vi "stop.vi"(8 "error in (no error)":errorcluster, 11 "TaskController in":refnum<class "TaskController.lvclass">) -> (0 "error out":errorcluster, 3 "TaskController out":refnum<class "TaskController.lvclass">)   [LabVIEW 2023, in "TLC_Daemon.lvlib" / "TaskController.lvclass"]
doc: "Stops the task (waits the task to finish executing).\n_____________________________________\nTLC Daemon 1.0.0.2\nCopyright (c) 2026 Andrea Cadei"
uses:
  TaskController.lvclass
  TaskController.lvclass/TaskController.ctl
  ITaskStopMechanism/ITaskStopMechanism.lvclass
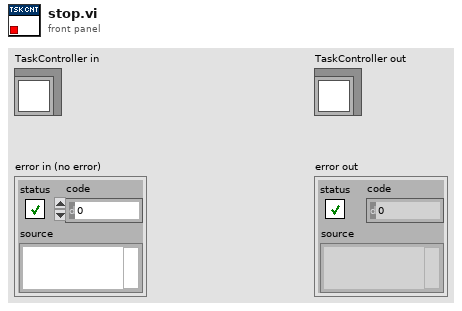
[diagram p1: front panel]
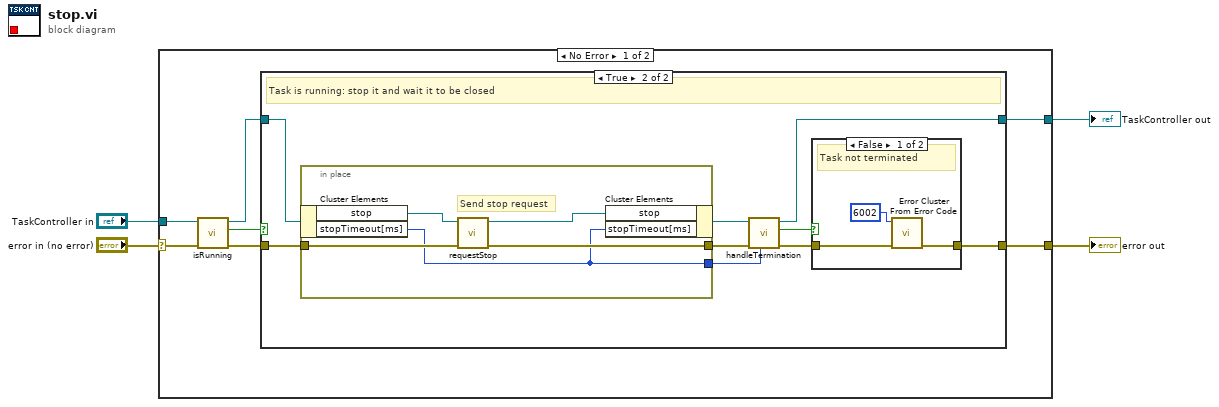
[diagram p0: block diagram]
diagram:
  n1 = case shown="No Error" "error in (no error)" {
    selector: "error in (no error)" -> [w7 w33]
    tunnel: [w10 w33] -> w3
    tunnel: [w11 w32] -> w1
    tunnel: "TaskController in" -> [w8 w32]
    frame No Error {
      n2 = call "isRunning.vi"("error in (no error)"=w7, "TaskController in"=w8) -> ("error out"=w6:errorcluster, "isRunning"=w5:bool, "TaskController out"=w9:refnum<class "TaskController.lvclass">)  [unwired: 7 in]
      n3 = case shown="True" w5 {
        tunnel: [w12 w18] -> w11
        tunnel: [w13 w14] -> w10
        tunnel: w9 -> [w12 w22]
        tunnel: w6 -> [w13 w21]
        frame False {
          # "Not running: do nothing"
        }
        frame True {
          # "Task is running: stop it and wait it to be closed"
          n4 = in-place {
            in-place-border: w21 -> [w31]
            in-place-border: [w30] -> w20
            in-place-border: [w27] -> w17
            # "Send stop request"
            n5 = in-place-cluster #1(w22) -> ("stop"=w29:refnum<class "ITaskStopMechanism.lvclass">, "stopTimeout[ms]"=w27:i32)
            n6 = call-dynamic "requestStop.vi"("error in (no error)"=w31, "ITaskStopMechanism in"=w29) -> ("error out"=w30:errorcluster, "ITaskStopMechanism out"=w28:refnum<class "ITaskStopMechanism.lvclass">)  [unwired: 8 in]
            n7 = in-place-cluster #1("stop"=w28, "stopTimeout[ms]"=w27) -> (w19:refnum<class "TaskController.lvclass">)
          }
          n8 = call "handleTermination.vi"("timeout[ms]"=w17, "error in (no error)"=w20, "TaskController in"=w19) -> ("error out"=w15:errorcluster, "terminated?"=w16:bool, "TaskController out"=w18:refnum<class "TaskController.lvclass">)  [unwired: 6 in]
          n9 = case shown="False" w16 {
            tunnel: w15 -> [w24 w26]
            tunnel: [w23 w26] -> w14
            frame False {
              # "Task not terminated"
              n10 = call <vilib>:"Error Cluster From Error Code.vi"("error in (no error)"=w24, "error code (0)"=6002) -> ("error out"=w23:errorcluster)  [unwired: 7 in]
            }
            frame True {
              # "Task terminated as expected"
            }
          }
        }
      }
    }
    frame Error {
    }
  }
  "error out" <- w3
  "TaskController out" <- w1
